vi "Read Prepend Minion ID.vi"(8 "error in (no error)":errorcluster, 11 "SystemLink configuration in":refnum<class "SystemLink configuration.lvclass">) -> (0 "error out":errorcluster, 2 "Prepend Minion ID":bool, 3 "SystemLink configuration out":refnum<class "SystemLink configuration.lvclass">)   [LabVIEW 2015, in "SystemLink configuration.lvclass"]
uses:
  SystemLink configuration.lvclass
  SystemLink configuration.lvclass/SystemLink configuration.ctl
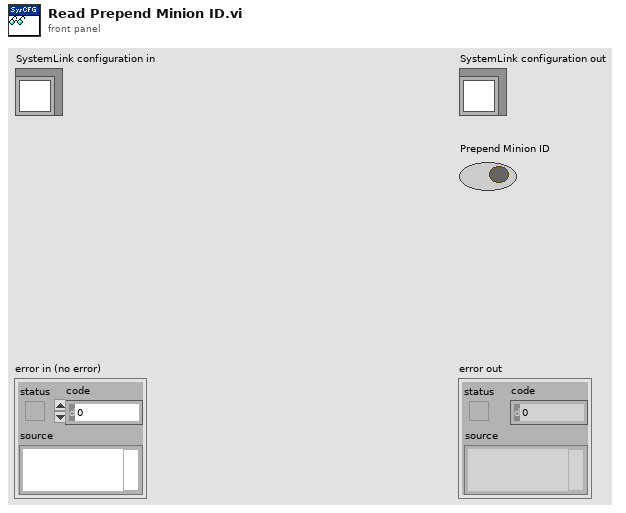
[diagram p1: front panel]
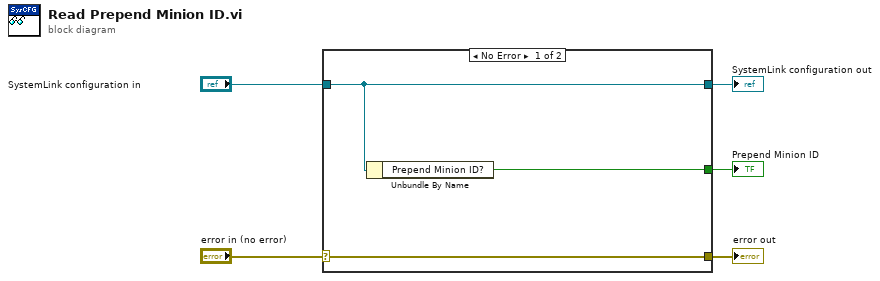
[diagram p0: block diagram]
diagram:
  n1 = case shown="No Error" "error in (no error)" {
    selector: "error in (no error)" -> [w8 w9]
    tunnel: [w8 w9] -> w4
    tunnel: [w7 w10] -> w2
    tunnel: "SystemLink configuration in" -> [w7 w10]
    tunnel: [w6 _] -> w1
    frame No Error {
      n2 = Unbundle By Name(w7) -> ("Prepend Minion ID?"=w6:bool)
    }
    frame Error {
    }
  }
  "error out" <- w4
  "SystemLink configuration out" <- w2
  "Prepend Minion ID" <- w1
